vi "Player Name.vi"(11 "Team":refnum<class "Team.lvclass">) -> (2 "Player Name":string)   [LabVIEW 2020, in "SquareBattle.lvlib" / "Team.lvclass"]
uses:
  Team.lvclass
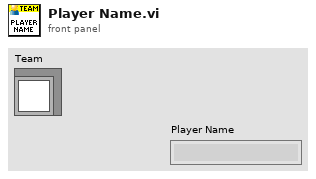
[diagram p1: front panel]
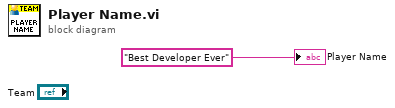
[diagram p0: block diagram]
diagram:
  "Player Name" <- "Best Developer Ever" ("Team Name")
